vi "Water Tank.vi"() -> (0 "Correct?":bool)   [LabVIEW 2013]
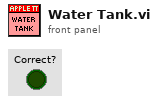
[diagram p1: front panel]
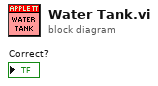
[diagram p0: block diagram]
diagram:
